vi "GEOM_SetWCSMod.vi"(10 "args in":string) -> (2 "response":string)   [LabVIEW 2016]
uses:
  GEOM_HeaderModule.ctl
  GEOM_VAR_action.ctl
panel:
  in  "HeaderModule":T1
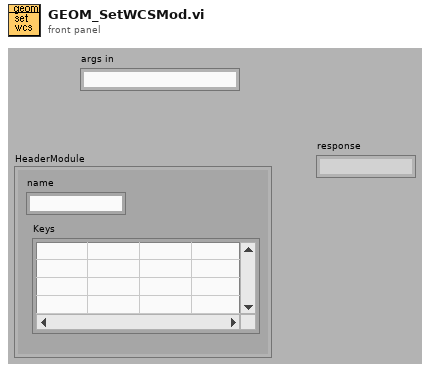
[diagram p1: front panel]
types:
  T1 = typedef "GEOM_HeaderModule.ctl" = cluster{"name":string, "Keys":string[][]}
  T2 = typedef "GEOM_VAR_action.ctl" = enum16{"read", "write"}
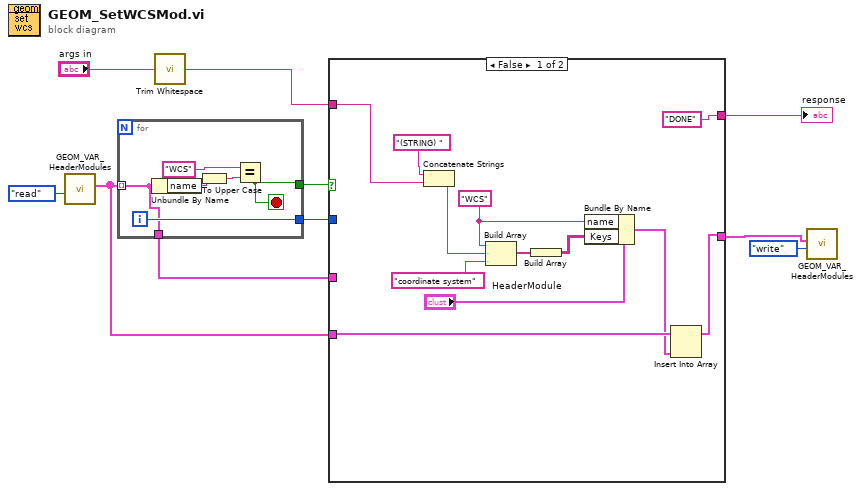
[diagram p0: block diagram]
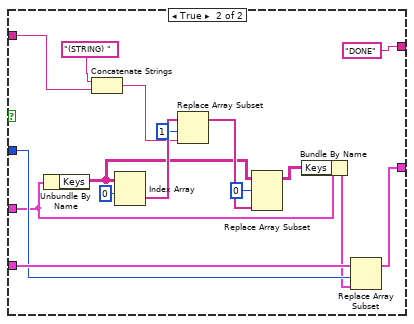
[diagram p2: hidden frame]
diagram:
  n1 = call "GEOM_VAR_HeaderModules.vi"("Action"=GEOM_VAR_action."read") -> ("GEOM_HeaderModules out"=w7:T1[])  [unwired: 1 in, 9 out]
  n2 = for {
    tunnel: w7 -> [w11] mode=indexing
    tunnel: [w13] -> w9
    tunnel: [w12] -> w8
    tunnel: [w11] -> w6
    i -> [w12]
    stop <- w13 stop-if-true
    n3 = Unbundle By Name(w11) -> ("name"=w16:string)
    n4 = To Upper Case(1:w16) -> (0:w14:string)
    n5 = Equal?(x="WCS", y=w14) -> (x = y?=w13:bool)
  }
  n6 = call <vilib>:"Trim Whitespace.vi"("string"="args in") -> ("trimmed string"=w1:string)  [unwired: 1 in]
  n7 = case shown="False" w9 {
    tunnel: w8 -> [_ w42]
    tunnel: w7 -> [w23 w43]
    tunnel: w6 -> [_ w39]
    tunnel: w1 -> [w18 w30]
    tunnel: [w21 w41] -> w4
    tunnel: ["DONE" ("response") "DONE" ("response")] -> w3
    frame False {
      w27 = "WCS" ("name")
      n8 = Concatenate Strings("(STRING) " ("format string"), w18) -> (w17:string)
      n9 = Build Array(w27, w17, "coordinate system" ("element")) -> (w25:string[])
      n10 = Build Array(w25) -> (w24:string[][])
      n11 = Bundle By Name(cluster="HeaderModule", "name"=w27, "Keys"=w24) -> (w22:T1)
      n12 = Insert Into Array(array=w23, new element=w22) -> (w21:T1[])  [unwired: 1 in]
    }
    frame True {
      n13 = Unbundle By Name(w39) -> ("Keys"=w33:string[][])
      n14 = Concatenate Strings("(STRING) " ("format string"), w30) -> (w29:string)
      n15 = Index Array(array=w33, index (row)=0) -> (element=w38:string[])  [unwired: 1 in]
      n16 = Replace Array Subset(array=w38, new element=w29, index=1) -> (w36:string[])
      n17 = Replace Array Subset(array=w33, new element=w36, index (row)=0 ("index")) -> (w32:string[][])  [unwired: 1 in]
      n18 = Bundle By Name(cluster=w39, "Keys"=w32) -> (w40:T1)
      n19 = Replace Array Subset(array=w43, new element=w40, index=w42) -> (w41:T1[])
    }
  }
  "response" <- w3
  n20 = call "GEOM_VAR_HeaderModules.vi"("Action"=GEOM_VAR_action."write", "GEOM_HeaderModules"=w4) -> ()  [unwired: 10 out]
